vi "Create Slave Instance (TCP).vi"(8 "error in (no error)":errorcluster, 9 "device data model":refnum<class "Device Data Model.lvclass">, 10 "port (502)":u16=502) -> (0 "error out":errorcluster, 3 "TCP slave instance":refnum<class "Modbus Slave.lvclass">)   [LabVIEW 2020, in "Modbus Slave.lvclass"]
doc: "Creates a serial or TCP Modbus slave instance. The Modbus slave instance you create includes a daemon. Daemon is a background process that responds to requests from Modbus master instances. You must manually select the polymorphic instance to use."
uses:
  <vilib>/Modbus/slave/Modbus Slave.lvclass
  C:/builds/penguin/iak/lvdsc/trunk/20.0/lv/vi.lib/Modbus/subvis/Modbus API/Modbus API.lvclass
  <vilib>/Modbus/subvis/Data and Functions/Device Data Model/Device Data Model.lvclass
  <vilib>/Modbus/subvis/Data and Functions/Standard Data Model/Standard Data Model.lvclass
  C:/builds/penguin/iak/lvdsc/trunk/20.0/lv/vi.lib/Modbus/subvis/Data and Functions/Device Data Model/Device Data Model.lvclass
  <vilib>/Modbus/subvis/Protocol/TCP/TCP Slave/TCP Slave.lvclass
  C:/builds/penguin/iak/lvdsc/trunk/20.0/lv/vi.lib/Modbus/subvis/Protocol/Interfaces/Network Slave/Network Slave.lvclass
  <vilib>/Modbus/subvis/Protocol/TCP/TCP Slave/TCP Slave.lvclass/TCP Slave.ctl
  <vilib>/Modbus/subvis/Transmission Data Unit (ADU)/IP Data Unit/IP Data Unit.lvclass
  C:/builds/penguin/iak/lvdsc/trunk/20.0/lv/vi.lib/Modbus/subvis/Transmission Data Unit (ADU)/Transmission Data Unit/Transmission Data Unit.lvclass
  <vilib>/Modbus/subvis/Transmission Data Unit (ADU)/Transmission Data Unit/Transmission Data Unit.lvclass/Transmission Data Unit.ctl
  <vilib>/Modbus/subvis/Data and Functions/Device Data Model/Device Data Model.lvclass/Device Data Model.ctl
  <vilib>/Modbus/slave/Modbus Slave.lvclass/Modbus Slave.ctl
  <vilib>/Modbus/subvis/Modbus API/Modbus API.lvclass/Modbus API.ctl
  <vilib>/Modbus/subvis/Protocol/TCP/TCP Slave/Accessors/port/Write Port.vi
  <vilib>/Modbus/subvis/Data and Functions/Device Data Model/Data Access/Initialized/Read Initialized.vi
  <vilib>/Utility/error.llb/Clear Errors.vi
  <vilib>/Modbus/subvis/Modbus API/Modbus API.lvclass
  <vilib>/Modbus/subvis/Transmission Data Unit (ADU)/Transmission Data Unit/Transmission Data Unit.lvclass
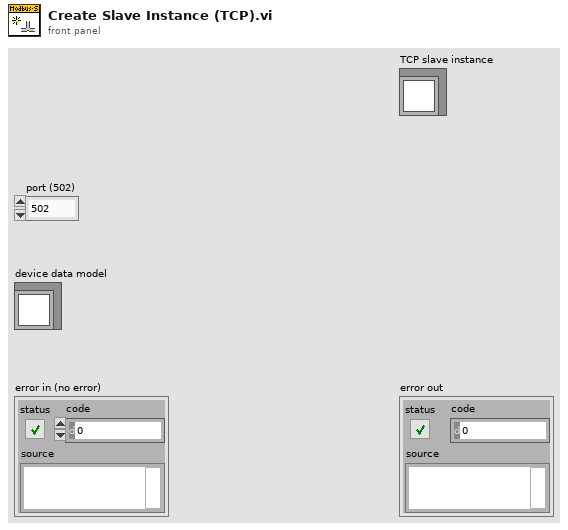
[diagram p1: front panel]
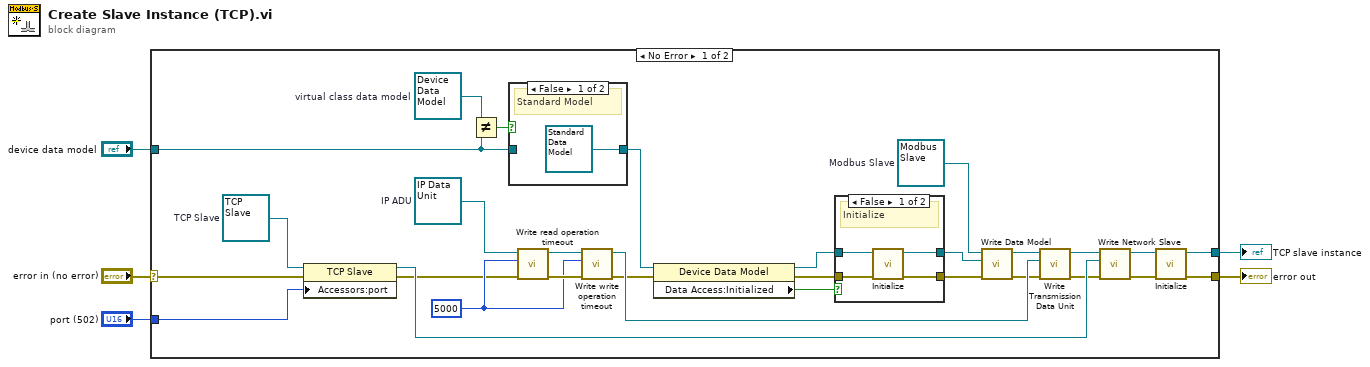
[diagram p0: block diagram]
diagram:
  n1 = case shown="No Error" "error in (no error)" {
    selector: "error in (no error)" -> [w6 w43]
    tunnel: "port (502)" -> [w33 _]
    tunnel: [w32 w43] -> w4
    tunnel: [w31 _] -> w3
    tunnel: "device data model" -> [w25 _]
    frame No Error {
      w27 = refnum<class "Device Data Model.lvclass"> refnum  # virtual class data model
      w16 = 5000 ("read operation timeout")
      w34 = refnum<class "TCP Slave.lvclass"> refnum  # TCP Slave
      w18 = refnum<class "IP Data Unit.lvclass"> refnum  # IP ADU
      w21 = refnum<class "Modbus Slave.lvclass"> refnum  # Modbus Slave
      n2 = property class="TCP Slave"(reference=w34, error in=w6, "Accessors:port"=w33) -> (reference out=w20:refnum<class "TCP Slave.lvclass">, error out=w8:errorcluster)
      n3 = Not Equal?(x=w27, y=w25) -> (x != y?=w26:bool)
      n4 = case shown="False" w26 {
        tunnel: w25 -> [_ w36]
        tunnel: [refnum<class "Standard Data Model.lvclass"> refnum ("Standard Data Model") w36] -> w24
        frame False {
          # "Standard Model"
        }
        frame True {
        }
      }
      n5 = call <vilib>:"Write read operation timeout.vi"("error in (no error)"=w8, "read operation timeout"=w16, "transmission data unit in"=w18) -> ("error out"=w19:errorcluster, "transmission data unit out"=w17:refnum<class "IP Data Unit.lvclass">)  [unwired: 7 in]
      n6 = call <vilib>:"Write write operation timeout.vi"("error in (no error)"=w19, "write operation timeout"=w16, "transmission data unit in"=w17) -> ("error out"=w7:errorcluster, "transmission data unit out"=w15:refnum<class "IP Data Unit.lvclass">)  [unwired: 7 in]
      n7 = property class="Device Data Model"(reference=w24, error in=w7) -> (reference out=w29:refnum<class "Device Data Model.lvclass">, error out=w30:errorcluster, "Data Access:Initialized"=w28:bool)
      n8 = case shown="False" w28 {
        tunnel: w30 -> [w40 w42]
        tunnel: [w39 w42] -> w22
        tunnel: [w38 w41] -> w23
        tunnel: w29 -> [w37 w41]
        frame False {
          # "Initialize"
          n9 = call-dynamic "Initialize.vi"("error in (no error)"=w40, "device data model in"=w37) -> ("error out"=w39:errorcluster, "device data model out"=w38:refnum<class "Device Data Model.lvclass">)  [unwired: 8 in]
        }
        frame True {
        }
      }
      n10 = call <vilib>:"Write Data Model.vi"("error in (no error)"=w22, "device data model"=w23, "Modbus slave in"=w21) -> ("error out"=w10:errorcluster, "Modbus slave out"=w14:refnum<class "Modbus Slave.lvclass">)  [unwired: 7 in]
      n11 = call <vilib>:"Write Transmission Data Unit.vi"("error in (no error)"=w10, "transmission data unit"=w15, "Modbus instance in"=w14) -> ("error out"=w11:errorcluster, "Modbus instance out"=w13:refnum<class "Modbus Slave.lvclass">)  [unwired: 7 in]
      n12 = call <vilib>:"Write Network Slave.vi"("error in (no error)"=w11, "network slave"=w20, "Modbus slave in"=w13) -> ("error out"=w9:errorcluster, "Modbus slave out"=w12:refnum<class "Modbus Slave.lvclass">)  [unwired: 7 in]
      n13 = call-dynamic "Initialize.vi"("error in (no error)"=w9, "Modbus slave in"=w12) -> ("error out"=w32:errorcluster, "Modbus slave out"=w31:refnum<class "Modbus Slave.lvclass">)  [unwired: 8 in]
    }
    frame Error {
    }
  }
  "error out" <- w4
  "TCP slave instance" <- w3
